vi "Wait or Write Status.vi"(11 "reach end":bool) -> (3 "Next Status":enum16{"Wait on Trigger", "Write DRAM"}(ring))   [LabVIEW 2015]
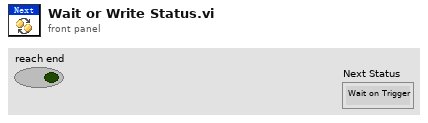
[diagram p1: front panel]
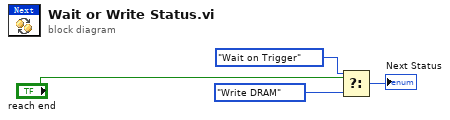
[diagram p0: block diagram]
diagram:
  n1 = Select(t=enum16{"Wait on Trigger", "Write DRAM"}."Wait on Trigger", s="reach end", f=enum16{"Wait on Trigger", "Write DRAM"}."Write DRAM") -> (s? t:f=→"Next Status":enum16{"Wait on Trigger", "Write DRAM"})
